vi "Generate missing time series header file.vi"(8 "error in (no error)":errorcluster, 11 "Timelapse data folder path":path) -> ()   [LabVIEW 2017]
uses:
  Functional Imaging Viewer/SubVIs/Experiment header interface/Typedefs/Header file interface module functions enum.ctl
  Globals/gl_Time series viewer globals.vi
panel:
  out "error out":errorcluster
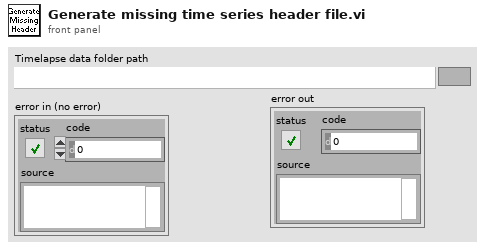
[diagram p1: front panel]
types:
  T1 = typedef "Header file interface module functions enum.ctl" = enum16{"Load experiment header file", "Save experiment header file", "Clear stored values", "Read stored values", "Update specific value in memory", "Update values in memory"}
  T2 = typedef "AVI playback header info cluster.ctl" = cluster{"Frame Size":u32, "AOD fill time (us)":dbl, "Dwell time (us)":dbl, "Frame period (ms)":dbl, "Number of Miniscans":u16, "Number of Pixels in Miniscan":u16}
  T3 = typedef "Header parameters cluster-ALL.ctl" = cluster{"LOGIN":T4, "GLOBAL PARAMETERS":T5, "IMAGING MODES":T7, "TIME SERIES":T8, "MOTOR Z-STACK ":T11, "AOL Z-STACK":T12, "FUNCTIONAL IMAGING":T13, "MOVEMENT CORRECTION":T17, "CALIBRATION":T19, "STATISTICS":T20, "BIOLOGY INFORMATION":T21}
  T4 = typedef "Header params -Login.ctl" = cluster{"User":string, "Profile":string, "Software Version":string, "Experiment Date Time":timestamp}
  T5 = typedef "Header params-Global Parameters.ctl" = cluster{"MicroscopeID":string, "Microscope Type":string, "Objective":string, "Field of View (um)":dbl, "Fill time (us)":dbl, "Experiment Type":T6, "Stimuli Trigger":bool, "Speed Logging":bool}
  T6 = typedef "Experiment Type.ctl" = enum16{"In vivo", "In vitro", "Testing", "Calibration", "Other"}
  T7 = typedef "Header params-Imaging Modes.ctl" = cluster{"Time Series":bool, "Motor Zstack":bool, "AOL Zstack":bool, "Functional Imaging":bool}
  T8 = typedef "Header params-Time Series.ctl" = cluster{"Basic Image meta data":T9, "AOL z":dbl}
  T9 = typedef "Header params-Basic image meta data.ctl" = cluster{"Wavelength (nm)":dbl, "# averaged frames":dbl, "laser power (%)":dbl, "Pockels":dbl, "pixel dwell time (us)":dbl, "pmt 1":dbl, "pmt 2":dbl, "back apperture":dbl, "zoom":dbl, "field of view":dbl, "Frame Size":T10, "AOL x centre":dbl, "AOL y centre":dbl, "Stage x position":dbl, "Stage y position":dbl, "Stage z position":dbl}
  T10 = typedef "Frame Size.ctl" = u16
  T11 = typedef "Header params-Motor Z-stack.ctl" = cluster{"Hdr Basic Image meta data":T9, "Z Start":dbl, "Z Stop":dbl, "No of Planes":i32}
  T12 = typedef "Header params-AOL Z-stack.ctl" = cluster{"Hdr Basic Image meta data":T9, "Z Start":dbl, "Z Stop":dbl, "No of Planes":i32}
  T13 = typedef "Header params-Functional Imaging.ctl" = cluster{"Functional Mode":T14, "Pockels Modulation":bool, "Number of pois":dbl, "Number of miniscans":dbl, "Number of cycles":dbl, "Number of trials":dbl, "Miniscan dwell time per pixel (us)":dbl, "Number of pixels in miniscan":dbl, "poi dwell time":dbl, "Rectangle ROI length":dbl, "Rectangle ROI height":dbl, "AOL Mode":T15, "Plane Mode":T16, "video length (sec)":dbl, "Frame rate (fps)":dbl, "Stimuli Timing (usec)":dbl, "Acquisition Length":dbl, "Basic Image meta data":T9, "Z Start (um)":dbl, "Z Stop (um)":dbl}
  T14 = typedef "Functional Mode.ctl" = enum16{"Point", "Line", "Patch", "Plane", "Volume"}
  T15 = typedef "AOL modes.ctl" = enum16{"Raster", "Structural", "Pointing", "Mini Scan", "Alignment"}
  T16 = typedef "Plane Mode.ctl" = u16
  T17 = typedef "Header params-Movement correction.ctl" = cluster{"Movement Correction":bool, "Axial Reference":bool, "Reference X Pixels":dbl, "Reference Y Pixels":dbl, "Reference Source":T18, "Reference dwell time (us)":dbl, "Number of Z lines":dbl, "Size of Z pixels":dbl, "Axial Pixels":dbl, "Reference Zoom":dbl, "Reference Average":dbl, "Proportional Scale":dbl, "Integral Scale":dbl, "Proportional Scale Z":dbl, "Integral Scale Z":dbl, "Scan Interval":dbl, "Ref Plot Refresh Rate":dbl}
  T18 = typedef "Reference source.ctl" = enum16{"Green channel", "Red channel"}
  T19 = typedef "Header params-Calibration Setup.ctl" = cluster{"Pockels Calibration File":path, "Calibration_ini file":path, "Setup_ini file":path}
  T20 = typedef "Header params-statistics.ctl" = cluster{"Z-stack duration (sec)":dbl, "Number of acquired data-points":dbl, "Acquisition time (ms)":dbl, "Number of acquired frames":dbl}
  T21 = typedef "Biology Information.ctl" = cluster{"Animal Code or Name":string, "Animal DoB":string, "Animal Age":string, "Animal Sex":string, "Animal Weight":string, "Date of Injection":string, "Date of Implant":string, "Site of Injection":string, "Animal Ear Notch":string, "AAV constructs":string, "Genetic background":string, "Optical reporter":string, "Region of brain imaged":string, "Other \ncomments":string}
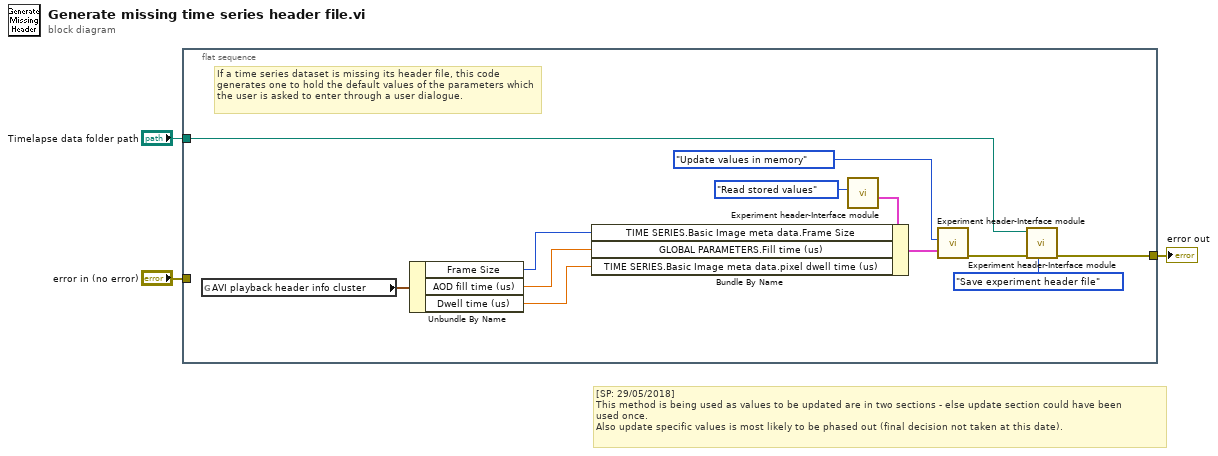
[diagram p0: block diagram]
diagram:
  # "[SP: 29/05/2018]\nThis method is being used as values to be updated are in two sections - else update section could have been\nused once.\nAlso update specific values is most likely to be phased out (final decision not taken at this date)."
  n1 = flat-sequence {
    tunnel: "error in (no error)" -> [_]
    tunnel: "Timelapse data folder path" -> [w13]
    tunnel: [w4] -> w1
    frame #0 {
      # "If a time series dataset is missing its header file, this code generates one to hold the default values of the parameters which the user is asked to enter through a user dialogue."
      n2 = global read "gl_Time series viewer globals.vi" "AVI playback header info cluster"() -> (w14:T2)
      n3 = Unbundle By Name(w14) -> ("Frame Size"=w10:u32, "AOD fill time (us)"=w9:dbl, "Dwell time (us)"=w8:dbl)
      n4 = call "Experiment header-Interface module.vi"("Function"=Header_file_interface_module_functions_enum."Read stored values") -> ("All header parameters out"=w11:T3)  [unwired: 9 in, 1 out]
      n5 = Bundle By Name(cluster=w11, "TIME SERIES.Basic Image meta data.Frame Size"=w10, "GLOBAL PARAMETERS.Fill time (us)"=w9, "TIME SERIES.Basic Image meta data.pixel dwell time (us)"=w8) -> (w6:T3)
      n6 = call "Experiment header-Interface module.vi"("All header parameters in"=w6, "Function"=Header_file_interface_module_functions_enum."Update values in memory") -> ("error out"=w5:errorcluster)  [unwired: 8 in, 1 out]
      n7 = call "Experiment header-Interface module.vi"("error in (no error)"=w5, "Function"=Header_file_interface_module_functions_enum."Save experiment header file", "Experiment data folder path"=w13) -> ("error out"=w4:errorcluster)  [unwired: 7 in, 1 out]
    }
  }
  "error out" <- w1
